vi "valves_large_liquid.vi"(0 "PID Gains Cluster Ref":refnum<vi>, 1 "Accept Autotune":bool, 2 "Controller Toggle (Manual Mode)":bool, 3 "Valve Manual Adjust":dbl, 5 "Slide Refnum in":refnum<vi>, 7 "file (use dialog)":path, 9 "Desired Setpoint":dbl, 11 "PID gains":T2, 12 "Current Process Variable Value":dbl, 13 "autotune? (F)":bool, 14 "Reinitialize Controller":bool) -> (4 "output to valve":dbl, 6 "output to slide":dbl, 8 "tuning completed?":bool, 10 "plant parameters out":T1, 15 "PID gains out":T2)   [LabVIEW 2017]
uses:
  <vilib>/addons/control/pid/autopid.llb/PID autotuning parameters (FO).ctl
  <vilib>/addons/control/pid/NI_PID_autopid.lvlib
panel:
  in  "threshold to lower gains":dbl=3.0
  in  "amount ot lower gains":dbl=100.0 format="%#_13g"
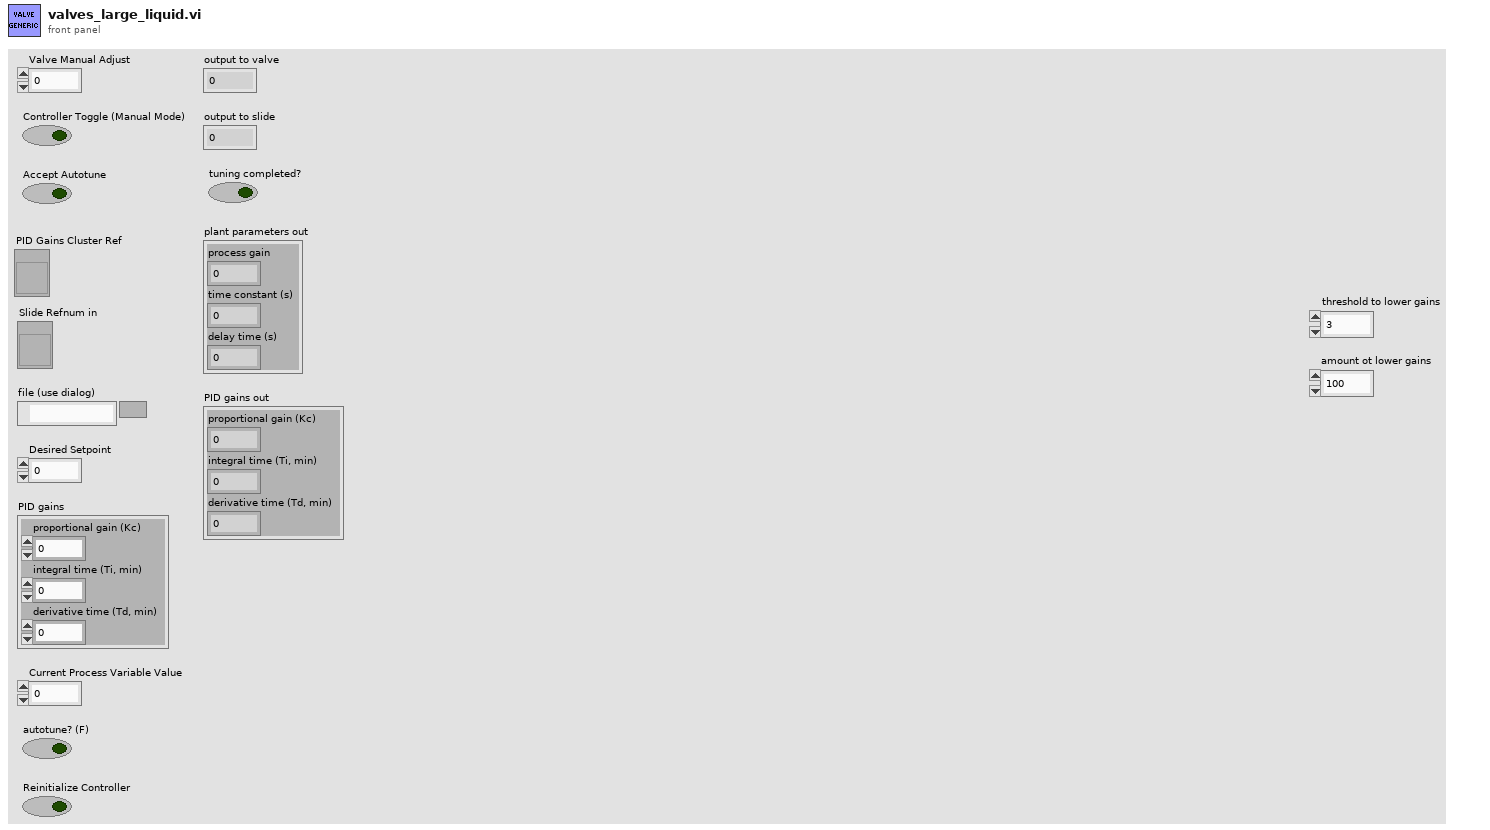
[diagram p1: front panel]
types:
  T1 = cluster{"process gain":dbl, "time constant (s)":dbl, "delay time (s)":dbl}
  T2 = cluster{"proportional gain (Kc)":dbl, "integral time (Ti, min)":dbl, "derivative time (Td, min)":dbl}
  T3 = typedef "NI_PID_autopid.lvlib/PID autotuning parameters (FO).ctl" = cluster{"type of controller":u16, "time constant factor":dbl, "step amplitude":dbl}
  T4 = enum8{"Enabled", "Disabled", "Disabled and Grayed Out"}
  T5 = cluster{dbl, "integral time (Ti, min)":dbl, "derivative time (Td, min)":dbl}
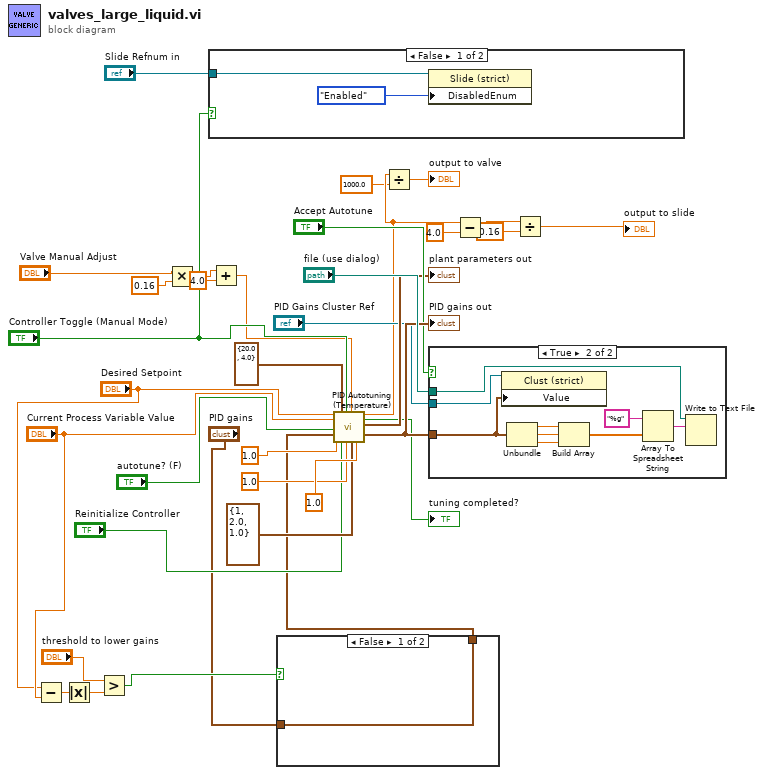
[diagram p0: block diagram]
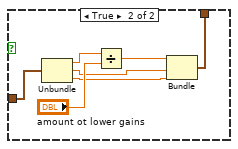
[diagram p2: hidden frame]
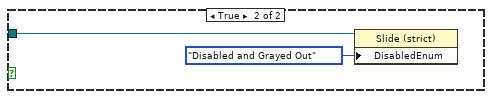
[diagram p4: hidden frame]
diagram:
  n1 = Subtract(x="Desired Setpoint", y="Current Process Variable Value") -> (x-y=w8:dbl)
  n2 = Absolute Value(x=w8) -> (abs(x)=w7:dbl)
  n3 = Greater?(x="threshold to lower gains", y=w7) -> (0:w5:bool)
  n4 = Multiply(x="Valve Manual Adjust", y=0.16) -> (x*y=w18:dbl)
  n5 = case shown="False" "Controller Toggle (Manual Mode)" {
    tunnel: "Slide Refnum in" -> [w36 w39]
    frame False {
      n6 = property on="Property Node" class="Slide (strict)"(reference=w36, "DisabledEnum"=T4."Enabled" ("Disabled")) -> ()  [unwired: 1 in, 2 out]
    }
    frame True {
      n7 = property on="Property Node" class="Slide (strict)"(reference=w39, "DisabledEnum"=T4."Disabled and Grayed Out" ("Disabled")) -> ()  [unwired: 1 in, 2 out]
    }
  }
  n8 = Add(x=w18, y=4.0) -> (x+y=w16:dbl)
  n9 = case shown="False" w5 {
    tunnel: "PID gains" -> [w40 w47]
    tunnel: [w40 w41] -> w3
    frame False {
    }
    frame True {
      n10 = Unbundle(w47) -> ("proportional gain (Kc)"=w46:dbl, "integral time (Ti, min)"=w43:dbl, "derivative time (Td, min)"=w42:dbl)
      n11 = Divide(x=w46, y="amount ot lower gains") -> (x/y=w44:dbl)
      n12 = Bundle(w44, "integral time (Ti, min)"=w43, "derivative time (Td, min)"=w42) -> (w41:T5)  [unwired: 1 in]
    }
  }
  n13 = call <vilib>:"PID Autotuning (Temperature).vi"("desired temperature"="Desired Setpoint", "measured temperature"="Current Process Variable Value", "autotune? (F)"="autotune? (F)", "PID gains in"=w3, "dt (s)"=1.0, "output range"=cluster{"output high":dbl, "output low":dbl} {"output high"=20.0, "output low"=4.0}, "reinitialize? (F)"="Reinitialize Controller", "auto? (T)"="Controller Toggle (Manual Mode)", "beta"=1.0, "manual control"=w16, "autotuning parameters"=T3 {"type of controller"=1, "time constant factor"=2.0, "step amplitude"=1.0}, "alpha"=1.0) -> ("output"=w10:dbl, "tuning completed?"=→"tuning completed?":bool, "plant parameters out"=→"plant parameters out":T1, "PID gains out"=w34:T2)  [unwired: 4 in]
  "PID gains out" <- w34
  n14 = Divide(x=w10, y=1000.0) -> (x/y=→"output to valve":dbl)
  n15 = case shown="True" "Accept Autotune" {
    tunnel: w34 -> [_ w56]
    tunnel: "file (use dialog)" -> [_ w49]
    tunnel: "PID Gains Cluster Ref" -> [_ w48]
    frame False {
    }
    frame True {
      n16 = property class="Clust (strict)"(reference=w48, "Value"=w56) -> ()  [unwired: 1 in, 2 out]
      n17 = Unbundle(w56) -> ("proportional gain (Kc)"=w55:dbl, "integral time (Ti, min)"=w54:dbl, "derivative time (Td, min)"=w53:dbl)
      n18 = Build Array(w55, w54, w53) -> (w52:dbl[])
      n19 = Array To Spreadsheet String(array=w52, 3:"%g" ("format string")) -> (spreadsheet string=w51:string)  [unwired: 1 in]
      n20 = Write to Text File(file (use dialog)=w49, text=w51) -> ()  [unwired: 2 in, 3 out]
    }
  }
  n21 = Subtract(x=w10, y=4.0) -> (x-y=w15:dbl)
  n22 = Divide(x=w15, y=0.16) -> (x/y=→"output to slide":dbl)
